vi "strain_gauge_start.vi"(8 "error in":errorcluster, 9 "Maximum Value":dbl=0.001, 10 "Minimum Value":dbl=-0.001, 11 "Physical Channel":tag="cDAQ4Mod1/ai0") -> (0 "error out":errorcluster, 3 "task out":refnum<k21>)   [LabVIEW 2022 SP3]
uses:
  <vilib>/DAQmx/create/channels.llb/DAQmx Create Channel (AI-Strain-Strain Gage).vi
  <vilib>/DAQmx/configure/timing.llb/DAQmx Timing (Sample Clock).vi
  <vilib>/DAQmx/calibration/calibrationInfo.llb/DAQmx Perform Shunt Calibration Ex (Strain).vi
panel:
  in  "Shunt Resistance":dbl=100000.0 format="%#.3p"
  in  "Shunt Element Location":i32(ring)=12465 caption="shunt element location" items=["R1"=12465, "R2"=12466, "R3"=12467, "R4"=14813, "None"=10230]
  in  "Sample Rate":dbl=1000.0
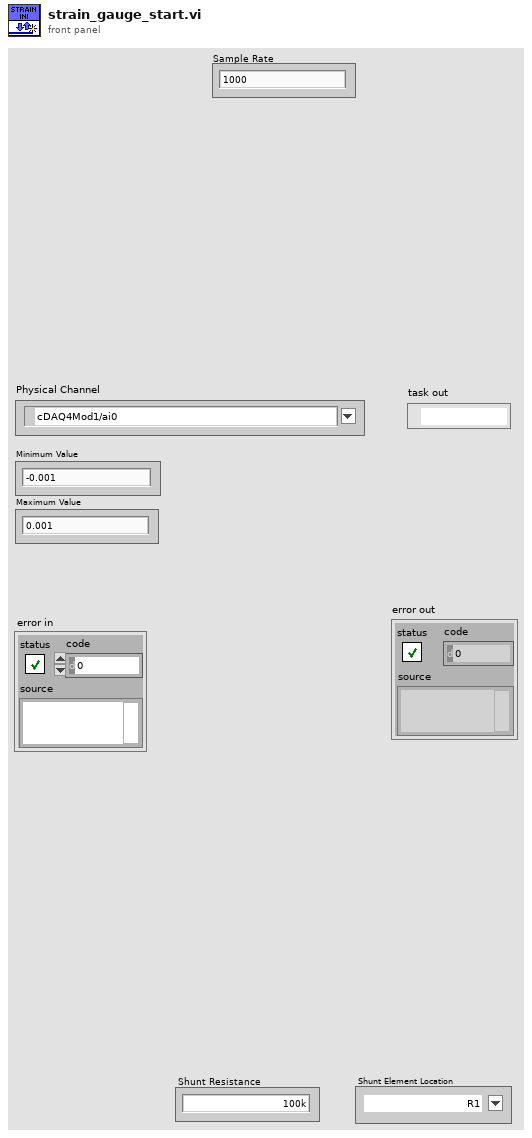
[diagram p1: front panel]
types:
  T1 = cluster{"Gage Factor":dbl, "Nominal Gage Resistance":dbl, "Poisson Ratio":dbl}
  T2 = cluster{"Strain Configuration":i32, "Lead Wire Resistance":dbl, "Initial Bridge Voltage":dbl, "Voltage Excitation Source":i32, "Voltage Excitation Value":dbl}
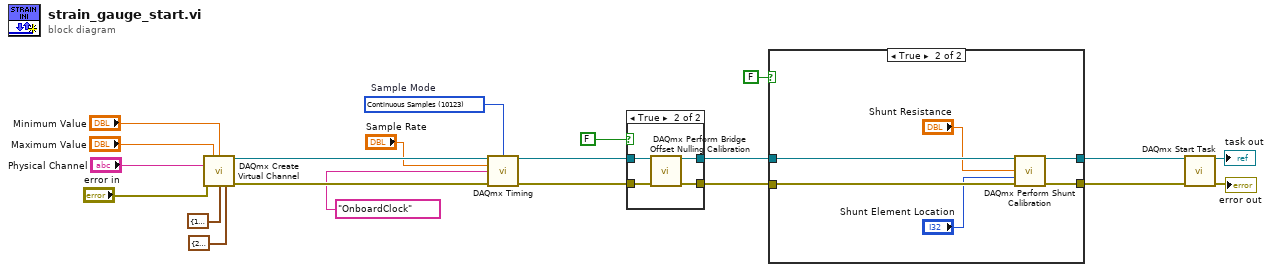
[diagram p0: block diagram]
diagram:
  w21 = 10123 items=["Finite Samples"=10178, "Continuous Samples"=10123, "Hardware Timed Single Point"=12522]  # Sample Mode
  n1 = call-poly <vilib>:"DAQmx Create Virtual Channel.vi"("maximum value"="Maximum Value", "minimum value"="Minimum Value", "physical channels"="Physical Channel", "error in"="error in", "bridge information"=T2 {"Strain Configuration"=10271, "Lead Wire Resistance"=0.0, "Initial Bridge Voltage"=0.0, "Voltage Excitation Source"=10200, "Voltage Excitation Value"=3.3} ("Bridge Information"), "strain gage information"=T1 {"Gage Factor"=2.0, "Nominal Gage Resistance"=350.0, "Poisson Ratio"=0.3} ("Strain Gage Information")) -> ("task out"=w19:refnum<k21>, "error out"=w20:errorcluster)  [unwired: 8 in]
  n2 = call-poly <vilib>:"DAQmx Timing.vi"("task/channels in"=w19, "sample mode"=w21, "rate"="Sample Rate", "source"=tag "OnboardClock" ("Sample Clock Source"), "error in"=w20) -> ("task out"=w5:refnum<k21>, "error out"=w4:errorcluster)  [unwired: 9 in]
  n3 = case shown="True" FALSE ("Do Offset Null?") {
    tunnel: [w23 w27] -> w10
    tunnel: [w22 w26] -> w9
    tunnel: w5 -> [w23 w25]
    tunnel: w4 -> [w22 w24]
    frame False {
    }
    frame True {
      n4 = call <vilib>:"DAQmx Perform Bridge Offset Nulling Calibration.vi"("task/channels in"=w25, "error in"=w24) -> ("task out"=w27:refnum<k21>, "error out"=w26:errorcluster)  [unwired: 12 in]
    }
  }
  n5 = case shown="True" FALSE ("Do Shunt Cal?") {
    tunnel: w10 -> [w29 w35]
    tunnel: w9 -> [w28 w34]
    tunnel: [w28 w33] -> w6
    tunnel: [w29 w32] -> w7
    frame False {
    }
    frame True {
      n6 = call-poly <vilib>:"DAQmx Perform Shunt Calibration.vi"("task/channels in"=w35, "shunt resistance"="Shunt Resistance", "shunt element location"="Shunt Element Location", "error in"=w34) -> ("task out"=w32:refnum<k21>, "error out"=w33:errorcluster)  [unwired: 10 in]
    }
  }
  n7 = call <vilib>:"DAQmx Start Task.vi"("task/channels in"=w7, "error in"=w6) -> ("task out"=→"task out":refnum<k21>, "error out"=→"error out":errorcluster)  [unwired: 12 in]
